vi "Configure Message.vi"(10 "Assert Data":T1) -> (3 "Input out":refnum<class "Input.lvclass">)   [LabVIEW 2016, in "AssertEngine.lvlib" / "Input.lvclass"]
uses:
  Input.lvclass
  Log Assert/Assert Data.ctl
  Input.lvclass/Input.ctl
  AssertEngine.lvlib
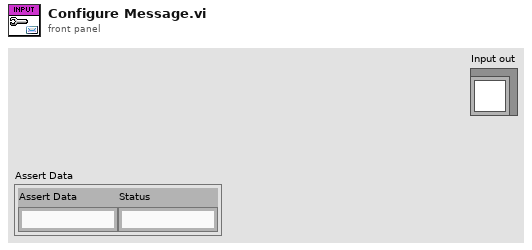
[diagram p1: front panel]
types:
  T1 = typedef "AssertEngine.lvlib/Assert Data.ctl" = cluster{"Assert Data":string, "Status":string}
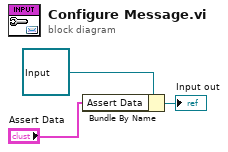
[diagram p0: block diagram]
diagram:
  n1 = Bundle By Name(cluster=refnum<class "Input.lvclass"> refnum ("Input in"), "Assert Data"="Assert Data") -> (→"Input out":refnum<class "Input.lvclass">)
